vi "Read Data.vi"(8 "error in (no error)":errorcluster, 11 "Readable in":refnum<class "Readable.lvclass">) -> (0 "error out":errorcluster, 1 "Channel Names":string[](array[string]), 2 "X array":T6, 3 "Readable out":refnum<class "Readable.lvclass">, 4 "Channel Units":string[](array[string]), 5 "Data Channels":T1, 7 "#Channels":i32)   [LabVIEW 2017, in "Readable.lvclass"]
doc: "Perform a measurement and return one or more channels of data. Public interface to \"_Read.vi.\" (Use this one!)"
uses:
  Readable.lvclass
  X array.ctl
  X.ctl
  Data Channels.ctl
  Data Channel.ctl
  Data Point.ctl
  Time.ctl
  Readable.lvclass/Readable.ctl
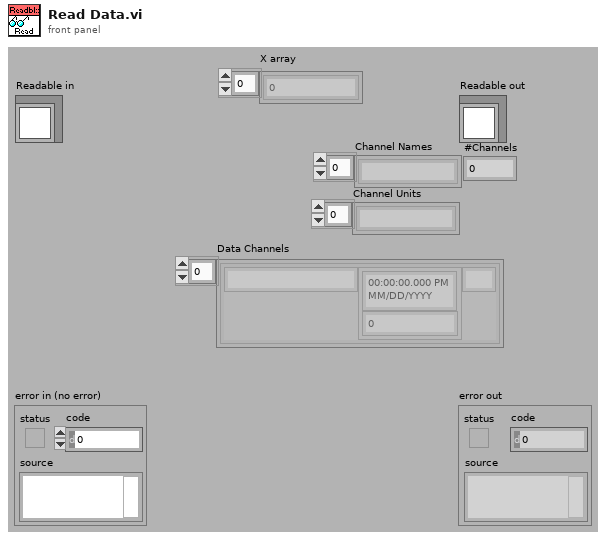
[diagram p1: front panel]
types:
  T1 = typedef "Readable.lvclass/Data Channels.ctl" = T2[]
  T2 = typedef "Readable.lvclass/Data Channel.ctl" = cluster{"Name":string, "Data Point":T3, "Unit":string}
  T3 = typedef "Readable.lvclass/Data Point.ctl" = cluster{"t":T4, "x":T5}
  T4 = typedef "Readable.lvclass/Time.ctl" = timestamp
  T5 = typedef "Readable.lvclass/X.ctl" = dbl
  T6 = typedef "Readable.lvclass/X array.ctl" = T5[]
  T7 = typedef "Readable.lvclass/Channel Units.ctl" = string[]
  T8 = typedef "Readable.lvclass/Channel Names.ctl" = string[]
  T9 = cluster{"seconds since 1Jan1904":timestamp, "x":T5}
  T10 = cluster{string, cluster{"seconds since 1Jan1904":timestamp, "x":T5}, "resulting string":string}
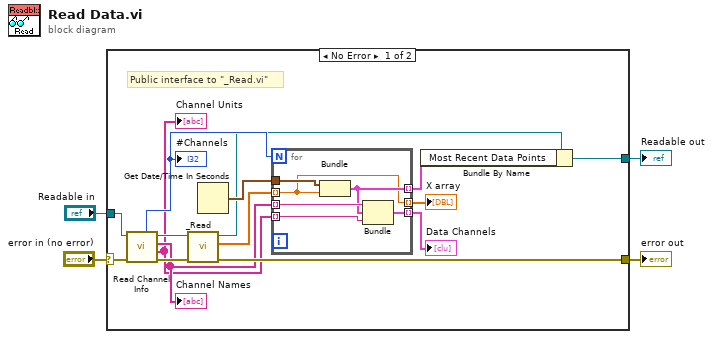
[diagram p0: block diagram]
diagram:
  n1 = case shown="No Error" "error in (no error)" {
    selector: "error in (no error)" -> [w16 w27]
    tunnel: [w19 w27] -> w3
    tunnel: [w10 w26] -> w1
    tunnel: "Readable in" -> [w18 w26]
    frame No Error {
      # "Public interface to \"_Read.vi\""
      n2 = call "Read Channel Info.vi"("error in (no error)"=w16, "Readable.lvclass in"=w18) -> ("error out"=w15:errorcluster, "Channel Units"=w7:T7, "Channel Names"=w8:T8, "Readable.lvclass out"=w17:refnum<class "Readable.lvclass">, "#Channels"=w13:i32)  [unwired: 5 in]
      "#Channels" <- w13
      "Channel Names" <- w8
      "Channel Units" <- w7
      n3 = call-dynamic "_Read.vi"("error in (no error)"=w15, "Readable in"=w17) -> ("error out"=w19:errorcluster, "X array"=w14:T6, "Readable out"=w11:refnum<class "Readable.lvclass">)  [unwired: 7 out]
      n4 = Get Date/Time In Seconds() -> (seconds since 1Jan1904=w12:timestamp)
      n5 = for {
        N: w13 -> [_]
        tunnel: w14 -> [w20] mode=indexing
        tunnel: w12 -> [w25]
        tunnel: [w23] -> w9 mode=indexing
        tunnel: w8 -> [w24] mode=indexing
        tunnel: w7 -> [w22] mode=indexing
        tunnel: [w21] -> w6 mode=indexing
        tunnel: [w20] -> w5 mode=indexing
        n6 = Bundle("seconds since 1Jan1904"=w25, "x"=w20) -> (w23:T9)  [unwired: 1 in]
        n7 = Bundle(w24, w23, "resulting string"=w22) -> (w21:T10)  [unwired: 1 in]
      }
      "X array" <- w5
      "Data Channels" <- w6
      n8 = Bundle By Name(cluster=w11, "Most Recent Data Points"=w9) -> (w10:refnum<class "Readable.lvclass">)
    }
    frame Error {
    }
  }
  "error out" <- w3
  "Readable out" <- w1
